vi "Connect.vi"(8 "error in":errorcluster, 10 "Additional Information":string, 11 "DB-MySQL in":refnum<class "DB-MySQL.lvclass">=refnum) -> (0 "error out":errorcluster, 3 "DB-MySQL out":refnum<class "DB-MySQL.lvclass">)   [LabVIEW 2014, in "hse-db.lvlib" / "DB-MySQL.lvclass"]
uses:
  DB-MySQL.lvclass
  DB-Interface.lvclass/DB-Interface.ctl
  DB-MySQL.lvclass/DB-MySQL.ctl
  DB-Interface.lvclass
  DB-Engines/MySQLTcp/MySQL (TCP).lvlib
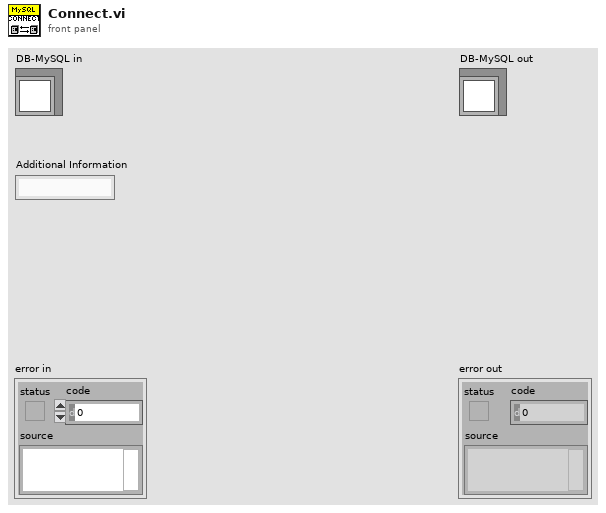
[diagram p1: front panel]
types:
  T1 = cluster{"User":string, "Password":string, "Database":string}
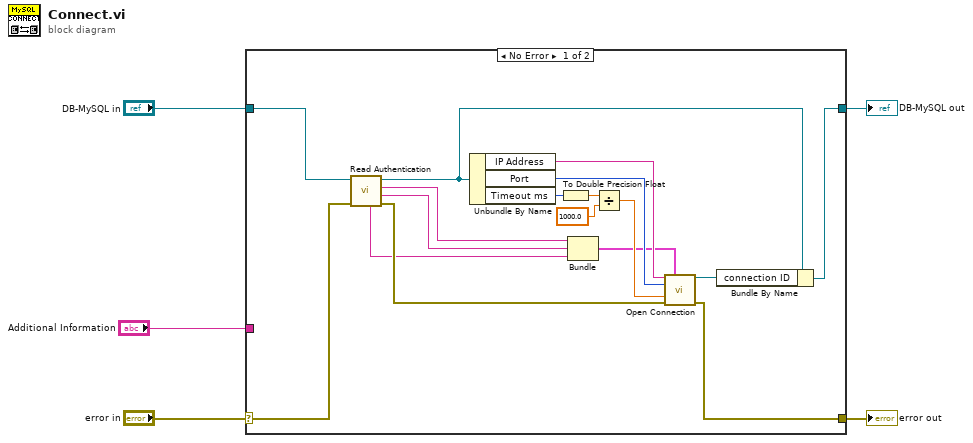
[diagram p0: block diagram]
diagram:
  n1 = case shown="No Error" "error in" {
    selector: "error in" -> [w21 w24]
    tunnel: [w17 w24] -> w4
    tunnel: [w22 w23] -> w2
    tunnel: "DB-MySQL in" -> [w20 w23]
    tunnel: "Additional Information" -> [_ _]
    frame No Error {
      n2 = call "Read Authentication.vi"("error in"=w21, "DB-Engine in"=w20) -> ("error out"=w18:errorcluster, "Password"=w8:string, "User"=w9:string, "DB-Engine out"=w19:refnum<class "DB-MySQL.lvclass">, "Database"=w7:string)  [unwired: 5 in]
      n3 = Unbundle By Name(w19) -> ("IP Address"=w15:string, "Port"=w14:u16, "Timeout ms"=w13:i32)
      n4 = To Double Precision Float(number=w13) -> (double precision float=w12:dbl)
      n5 = Bundle("User"=w9, "Password"=w8, "Database"=w7) -> (w6:T1)  [unwired: 1 in]
      n6 = Divide(x=w12, y=1000.0) -> (x/y=w10:dbl)
      n7 = call "Open Connection.vi"("Server Address"=w15, "Authentication"=w6, "Port (3306)"=w14, "timeout (15s)"=w10, "error in (no error)"=w18) -> ("connection ID out"=w16:refnum<k5>, "error out"=w17:errorcluster)  [unwired: 9 in]
      n8 = Bundle By Name(cluster=w19, "connection ID"=w16) -> (w22:refnum<class "DB-MySQL.lvclass">)
    }
    frame Error {
    }
  }
  "error out" <- w4
  "DB-MySQL out" <- w2
